vi "Set ParameterName.vi"(8 "error in":errorcluster, 10 "ParameterName":refnum<class "Value.lvclass">, 11 "Object Type in":refnum<class "Object Type Base.lvclass">) -> (0 "error out":errorcluster, 3 "Object Type out":refnum<class "Object Type Base.lvclass">)   [LabVIEW 2024, in "Electronic Datasheet.lvlib" / "Object Type Base.lvclass"]
uses:
  Object Type Base.lvclass
  Object Type Base.lvclass/Object Type Base.ctl
  Value/Value.lvclass
  Electronic Datasheet.lvlib
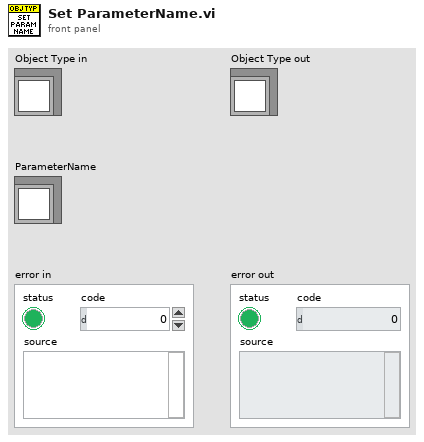
[diagram p1: front panel]
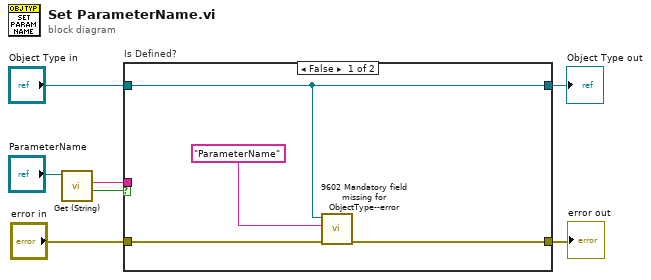
[diagram p0: block diagram]
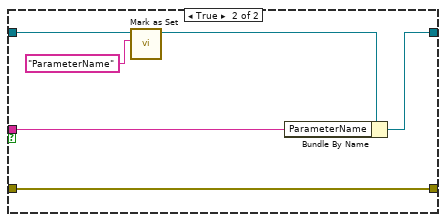
[diagram p2: hidden frame]
diagram:
  n1 = call "Get (String).vi"("Value in"="ParameterName") -> ("Defined?"=w4:bool, "Value"=w3:string)  [unwired: 8 in, 1 out]
  n2 = case "Is Defined?" shown="False" w4 {
    tunnel: [w8 w17] -> w7
    tunnel: "Object Type in" -> [w8 w16]
    tunnel: w3 -> [_ w13]
    tunnel: "error in" -> [w11 w12]
    tunnel: [w10 w12] -> w1
    frame False {
      n3 = call "9602 Mandatory field missing for ObjectType--error.vi"("error in"=w11, "Field Name"="ParameterName" ("error message (\"\")"), "Object Type Base"=w8) -> ("error out"=w10:errorcluster)  [unwired: 8 in]
    }
    frame True {
      n4 = call "Mark as Set.vi"("Field name"="ParameterName", "Object Type in"=w16) -> ("Object Type out"=w15:refnum<class "Object Type Base.lvclass">)  [unwired: 9 in]
      n5 = Bundle By Name(cluster=w15, "ParameterName"=w13) -> (w17:refnum<class "Object Type Base.lvclass">)
    }
  }
  "Object Type out" <- w7
  "error out" <- w1
